vi "Lab13_LabView.vi"() -> ()   [LabVIEW 2022 SP3]
uses:
  <vilib>/Instr/_visa.llb/VISA Configure Serial Port (Instr).vi
panel:
  out "LED 6":bool
  out "LED 5":bool
  out "LED 4":bool
  out "LED 3":bool
  out "LED 2":bool
  out "LED 1":bool
  in  "VISA resource name":refnum<visa-resource-name>
  in  "Switch 1":bool
  in  "Switch 2":bool
  in  "stop":bool
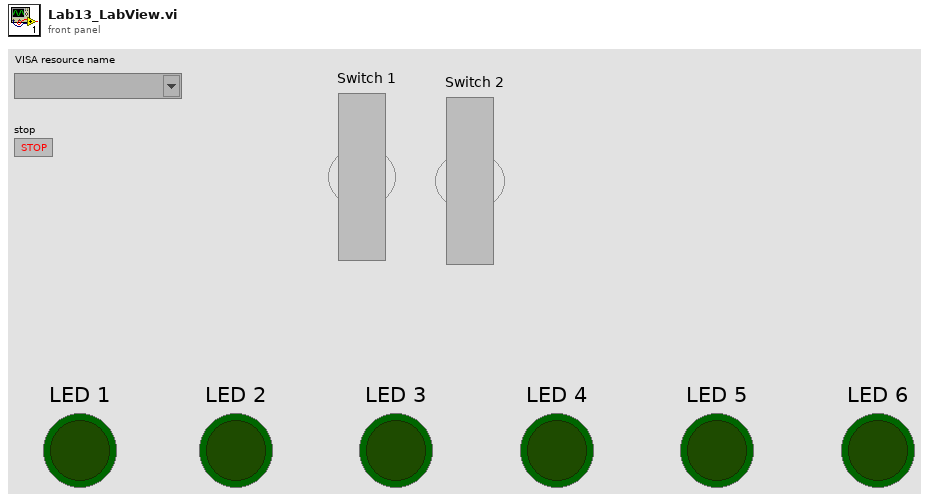
[diagram p1: front panel]
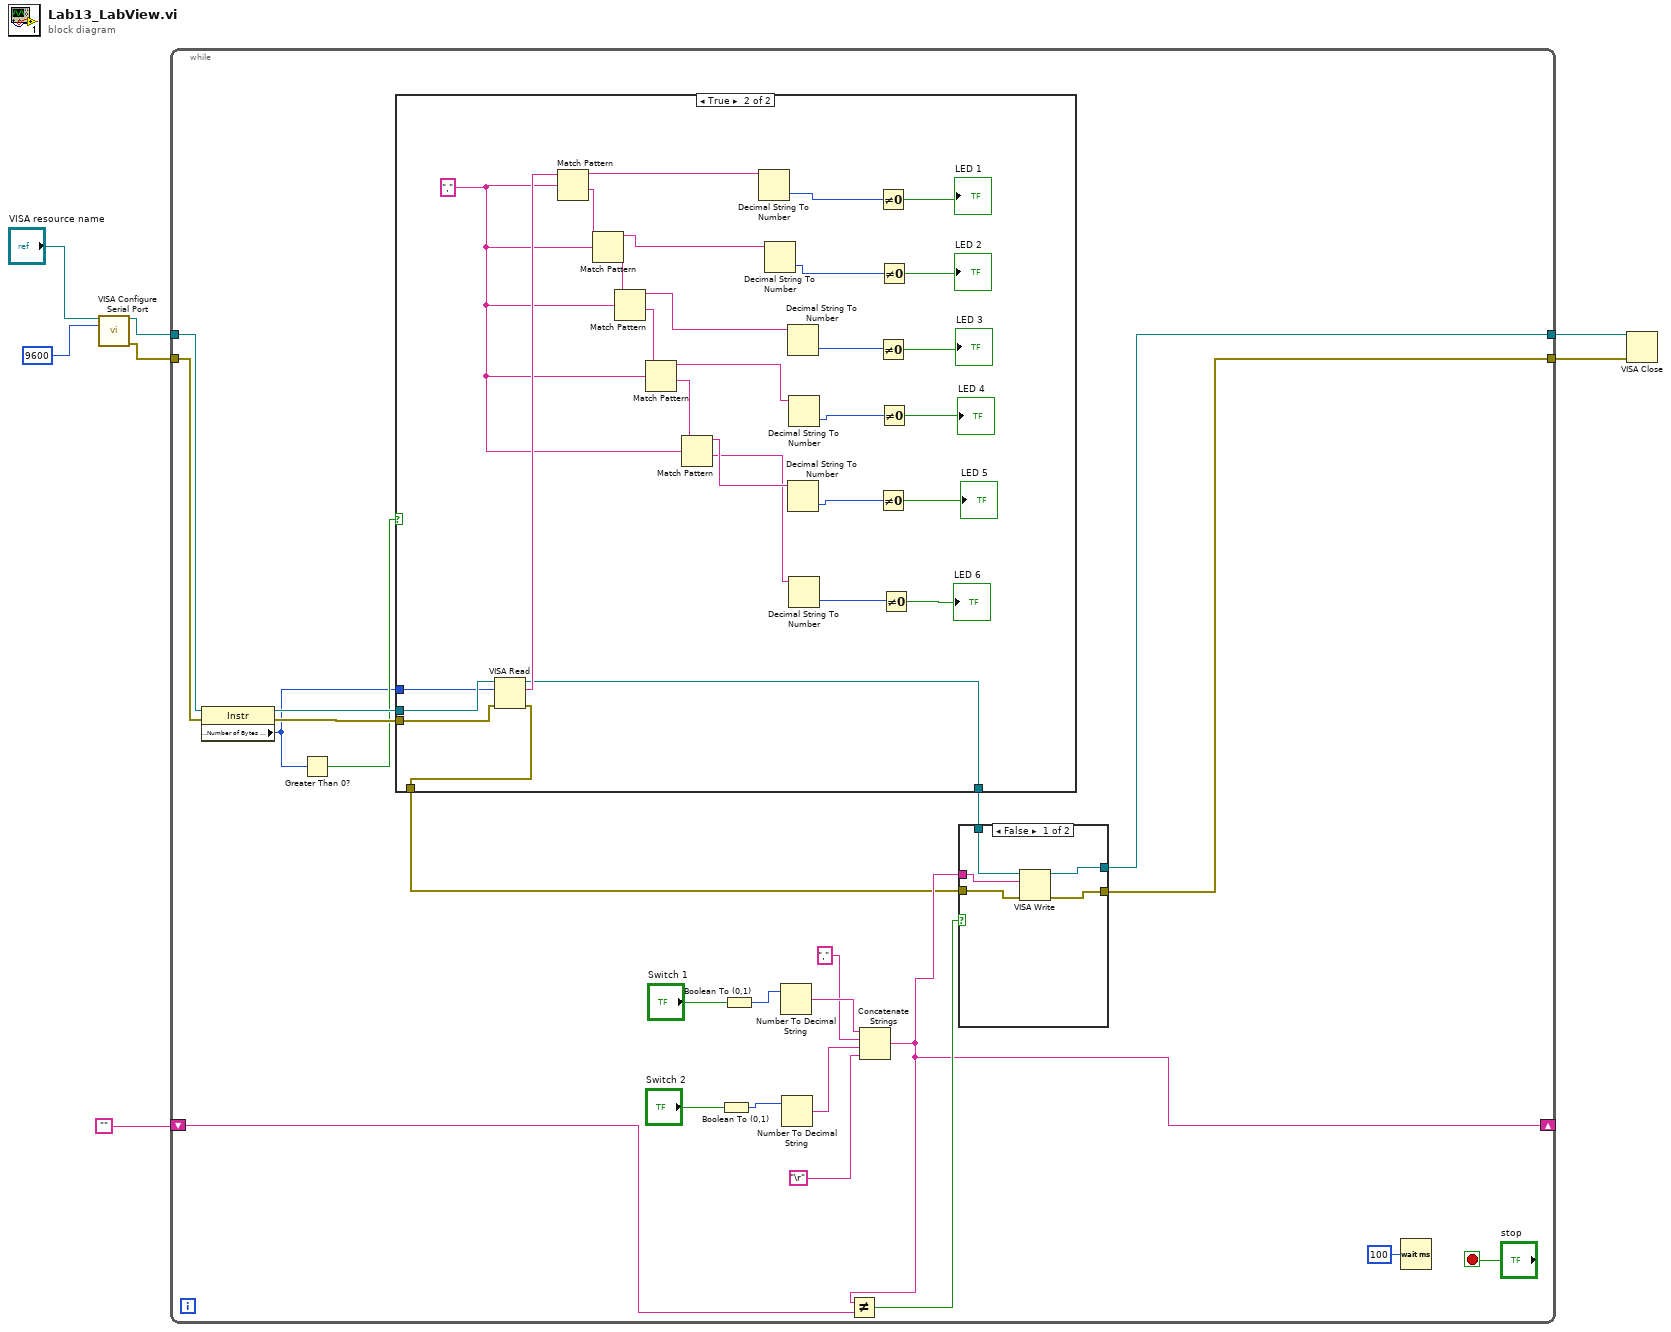
[diagram p0: block diagram]
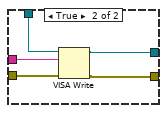
[diagram p3: hidden frame]
diagram:
  n1 = call-poly "VISA Configure Serial Port"("VISA resource name"="VISA resource name", "baud rate (9600)"=u32 9600) -> ("VISA resource name out"=w7:refnum<visa-resource-name>, "error out"=w6:errorcluster)  [unwired: 12 in]
  n2 = while {
    tunnel: w7 -> [w10]
    tunnel: w6 -> [w9]
    tunnel: [w21] -> w3
    tunnel: [w22] -> w2
    shift-right: [w18] -> _
    shift-left: "" -> [w20]
    stop <- "stop" stop-if-true
    n3 = property class="Instr"(reference=w10, error in=w9) -> (reference out=w15:refnum<visa-resource-name>, error out=w14:errorcluster, "Serial Settings:Number of Bytes at Serial Port"=w11:u32)
    n4 = Greater Than 0?(x=w11) -> (x > 0?=w13:bool)
    n5 = case shown="True" w13 {
      tunnel: w15 -> [w31 w61]
      tunnel: w14 -> [w32 w60]
      tunnel: [w32 w59] -> w12
      tunnel: w11 -> [_ w58]
      tunnel: [w31 w33] -> w8
      frame False {
      }
      frame True {
        w35 = ","
        n6 = VISA Read(VISA resource name=w61, byte count=w58, error in (no error)=w60) -> (VISA resource name out=w33:refnum<visa-resource-name>, read buffer=w57:string, error out=w59:errorcluster)  [unwired: 1 out]
        n7 = Match Pattern(string=w57, regular expression=w35) -> (before substring=w49:string, after substring=w48:string)  [unwired: 1 in, 2 out]
        n8 = Match Pattern(string=w48, regular expression=w35) -> (before substring=w46:string, after substring=w41:string)  [unwired: 1 in, 2 out]
        n9 = Match Pattern(string=w41, regular expression=w35) -> (before substring=w40:string, after substring=w39:string)  [unwired: 1 in, 2 out]
        n10 = Match Pattern(string=w39, regular expression=w35) -> (before substring=w37:string, after substring=w38:string)  [unwired: 1 in, 2 out]
        n11 = Match Pattern(string=w38, regular expression=w35) -> (before substring=w36:string, after substring=w34:string)  [unwired: 1 in, 2 out]
        n12 = Decimal String To Number(string=w49) -> (number=w50:i32)  [unwired: 2 in, 1 out]
        n13 = Decimal String To Number(string=w46) -> (number=w47:i32)  [unwired: 2 in, 1 out]
        n14 = Decimal String To Number(string=w40) -> (number=w45:i32)  [unwired: 2 in, 1 out]
        n15 = Decimal String To Number(string=w36) -> (number=w43:i32)  [unwired: 2 in, 1 out]
        n16 = Decimal String To Number(string=w37) -> (number=w44:i32)  [unwired: 2 in, 1 out]
        n17 = Decimal String To Number(string=w34) -> (number=w42:i32)  [unwired: 2 in, 1 out]
        n18 = Not Equal To 0?(x=w50) -> (x != 0?=→"LED 1":bool)
        n19 = Not Equal To 0?(x=w45) -> (x != 0?=→"LED 3":bool)
        n20 = Not Equal To 0?(x=w43) -> (x != 0?=→"LED 5":bool)
        n21 = Not Equal To 0?(x=w47) -> (x != 0?=→"LED 2":bool)
        n22 = Not Equal To 0?(x=w44) -> (x != 0?=→"LED 4":bool)
        n23 = Not Equal To 0?(x=w42) -> (x != 0?=→"LED 6":bool)
      }
    }
    n24 = Boolean To (0,1)(Boolean="Switch 2") -> (0, 1=w29:i16)
    n25 = Boolean To (0,1)(Boolean="Switch 1") -> (0, 1=w30:i16)
    n26 = Number To Decimal String(number=w30) -> (decimal integer string=w26:string)  [unwired: 1 in]
    n27 = Number To Decimal String(number=w29) -> (decimal integer string=w25:string)  [unwired: 1 in]
    n28 = Concatenate Strings(w26, ",", w25, "\r") -> (w18:string)
    n29 = Not Equal?(x=w18, y=w20) -> (x != y?=w19:bool)
    n30 = case shown="False" w19 {
      tunnel: [w64 w71] -> w22
      tunnel: [w63 w70] -> w21
      tunnel: w18 -> [w62 w69]
      tunnel: w12 -> [w65 w68]
      tunnel: w8 -> [w66 w67]
      frame False {
        n31 = VISA Write(VISA resource name=w66, write buffer=w62, error in (no error)=w65) -> (VISA resource name out=w64:refnum<visa-resource-name>, error out=w63:errorcluster)  [unwired: 1 out]
      }
      frame True {
        n32 = VISA Write(VISA resource name=w67, write buffer=w69, error in (no error)=w68) -> (VISA resource name out=w71:refnum<visa-resource-name>, error out=w70:errorcluster)  [unwired: 1 out]
      }
    }
    n33 = Wait (ms)(milliseconds to wait=u32 100) -> ()  [unwired: 1 out]
  }
  n34 = VISA Close(VISA resource name=w2, error in (no error)=w3) -> ()  [unwired: 1 out]
